vi "SequenceEvent.ExecuteCompleted.vi"(4 "Test Result":refnum<user-event>, 5 "Event Data":cluster{"sender":refnum<k24>, "e":refnum<k24>}, 6 "Control Ref":refnum<k24>, 7 "Event Common Data":T1) -> ()   [LabVIEW 2015, in "Simple Sequence Tools - Execution.lvlib"]
uses:
  Simple Sequence Tools - Execution.lvlib
  NationalInstruments.VeriStand.RealTimeSequenceDefinitionApi
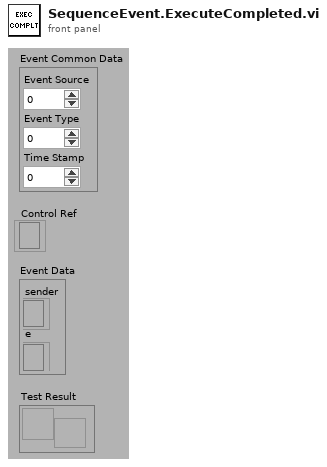
[diagram p1: front panel]
types:
  T1 = cluster{"Event Source":i32, "Event Type":u32, "Time Stamp":u32}
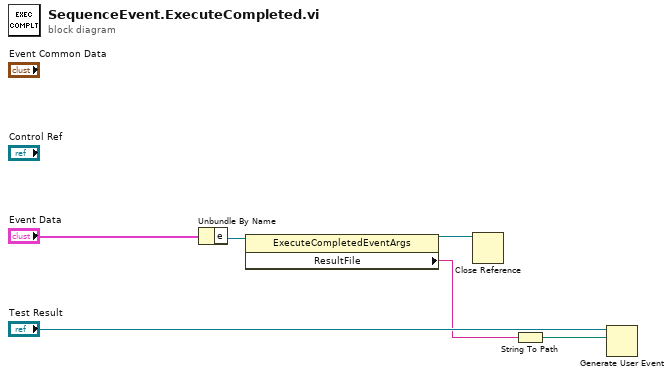
[diagram p0: block diagram]
diagram:
  n1 = Unbundle By Name("Event Data") -> ("e"=w5:refnum<k24>)
  n2 = property class="ExecuteCompletedEventArgs"(reference=w5) -> (reference out=w4:refnum<k24>, "ResultFile"=w3:string)  [unwired: 1 in, 1 out]
  n3 = Close Reference(reference=w4) -> ()  [unwired: 1 in, 1 out]
  n4 = String To Path(string=w3) -> (path=w2:path)
  n5 = Generate User Event(user event="Test Result", event data cluster=w2) -> ()  [unwired: 2 in, 2 out]
